vi "Filtro_derivadas(SubVI).vi"(11 "Pitch DMARS":dbl) -> (1 "Second derivative":dbl, 2 "First derivative":dbl, 3 "Filtered x":dbl)   [LabVIEW 2017]
uses:
  <vilib>/Analysis/3filter.llb/Filter Passband Type.ctl
  <vilib>/ptbypt/NI_PtbyPt.lvlib
  <vilib>/Analysis/NI_AALBase.lvlib
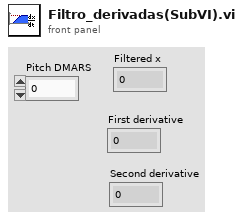
[diagram p1: front panel]
types:
  T1 = typedef "NI_AALBase.lvlib/Filter Passband Type.ctl" = enum32{"Lowpass", "Highpass", "Bandpass", "Bandstop"}
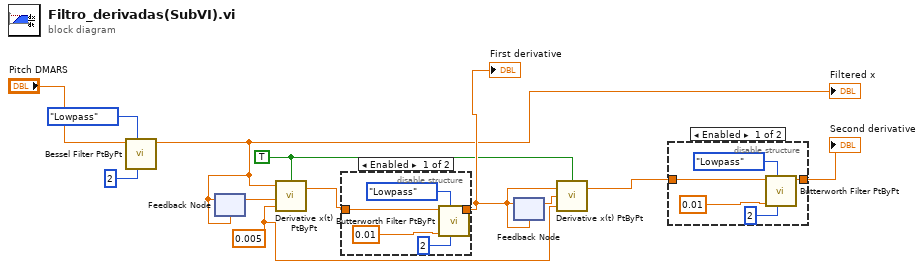
[diagram p0: block diagram]
diagram:
  w7 = 0.005 ("dt")
  w3 = TRUE ("initialize")
  n1 = call <vilib>:"Bessel Filter PtByPt.vi"("order"=2, "filter type"=Filter_Passband_Type."Lowpass", "x"="Pitch DMARS") -> ("Filtered x"=w4:dbl)  [unwired: 6 in, 1 out]
  "Filtered x" <- w4
  n2 = feedback #1(w4) -> (w5:dbl)
  n3 = feedback-in #1(w4) -> ()
  n4 = call <vilib>:"Derivative x(t) PtByPt.vi"("initialize"=w3, "dt"=w7, "initial condition"=w5, "x"=w4) -> ("dx/dt"=w11:dbl)  [unwired: 1 out]
  n5 = disable-structure shown="Enabled" {
    disable-tunnel: w11 -> [w15 w18]
    disable-tunnel: [w13 w18] -> w8
    frame Enabled {
      n6 = call <vilib>:"Butterworth Filter PtByPt.vi"("order"=2, "filter type"=Filter_Passband_Type."Lowpass", "low cutoff freq: fl"=0.01 ("high cutoff freq: fh"), "x"=w15) -> ("Filtered x"=w13:dbl)  [unwired: 5 in, 1 out]
    }
    frame Disabled {
    }
  }
  "First derivative" <- w8
  n7 = feedback #2(w8) -> (w6:dbl)
  n8 = feedback-in #2(w8) -> ()
  n9 = call <vilib>:"Derivative x(t) PtByPt.vi"("initialize"=w3, "dt"=w7, "initial condition"=w6, "x"=w8) -> ("dx/dt"=w10:dbl)  [unwired: 1 out]
  n10 = disable-structure shown="Enabled" {
    disable-tunnel: w10 -> [w21 w24]
    disable-tunnel: [w19 w24] -> w12
    frame Enabled {
      n11 = call <vilib>:"Butterworth Filter PtByPt.vi"("order"=2, "filter type"=Filter_Passband_Type."Lowpass", "low cutoff freq: fl"=0.01 ("high cutoff freq: fh"), "x"=w21) -> ("Filtered x"=w19:dbl)  [unwired: 5 in, 1 out]
    }
    frame Disabled {
    }
  }
  "Second derivative" <- w12
